vi "Read Object Coordinates.vi"(8 "error in (no error)":errorcluster, 11 "Pane Object Position in":refnum<class "Pane Object Position.lvclass">) -> (0 "error out":errorcluster, 2 "Object Coordinates":T1, 3 "Pane Object Position out":refnum<class "Pane Object Position.lvclass">)   [LabVIEW 2018, in "Pane Object Position.lvclass"]
uses:
  Pane Object Position.lvclass
  Object Coordinates.ctl
  Pane Object Position.lvclass/Pane Object Position.ctl
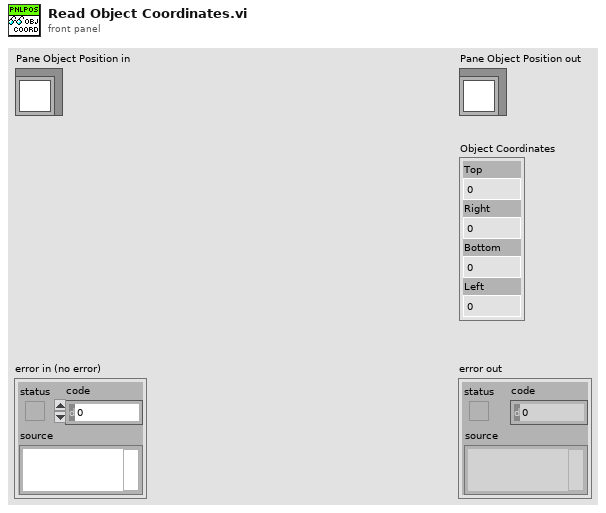
[diagram p1: front panel]
types:
  T1 = typedef "Pane Object Position.lvclass/Object Coordinates.ctl" = cluster{"Top":i32, "Right":i32, "Bottom":i32, "Left":i32}
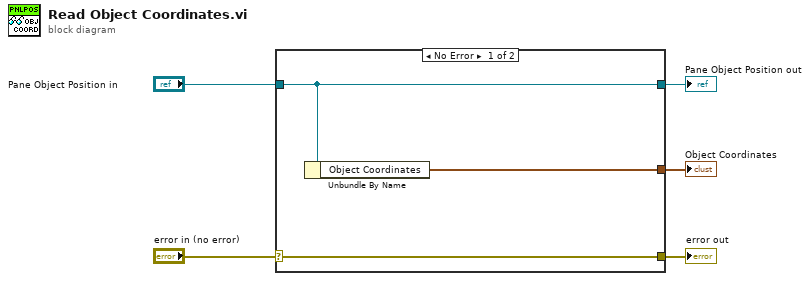
[diagram p0: block diagram]
diagram:
  n1 = case shown="No Error" "error in (no error)" {
    selector: "error in (no error)" -> [w8 w9]
    tunnel: [w8 w9] -> w4
    tunnel: [w7 w10] -> w2
    tunnel: "Pane Object Position in" -> [w7 w10]
    tunnel: [w6 _] -> w1
    frame No Error {
      n2 = Unbundle By Name(w7) -> ("Object Coordinates"=w6:T1)
    }
    frame Error {
    }
  }
  "error out" <- w4
  "Pane Object Position out" <- w2
  "Object Coordinates" <- w1
